vi "Base64 From Base64-URL.vi"(11 "Base64-URL String":string) -> (3 "Base64 String":string)   [LabVIEW 2018, in "Base64.lvlib"]
uses:
  Base64.lvlib
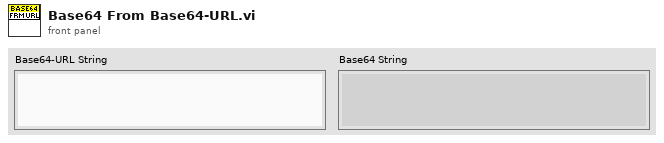
[diagram p1: front panel]
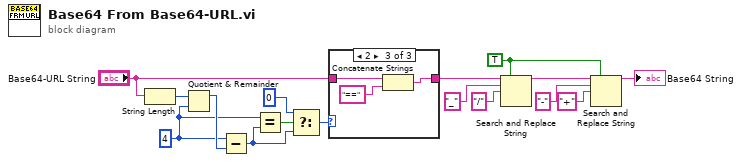
[diagram p0: block diagram]
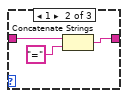
[diagram p3: hidden frame]
diagram:
  w3 = TRUE ("replace all? (F)")
  w14 = 4 ("y")
  n1 = String Length(string="Base64-URL String") -> (length=w16:i32)
  n2 = Quotient & Remainder(x=w16, y=w14) -> (x-y*floor(x/y)=w15:i32)  [unwired: 1 out]
  n3 = Subtract(x=w14, y=w15) -> (x-y=w12:i32)
  n4 = Equal?(x=w14, y=w12) -> (x = y?=w13:bool)
  n5 = Select(t=0, s=w13, f=w12) -> (s? t:f=w10:i32)
  n6 = case shown="2" w10 {
    tunnel: "Base64-URL String" -> [w17 w20 w23]
    tunnel: [w17 w18 w21] -> w2
    frame Default {
    }
    frame 1 {
      n7 = Concatenate Strings(w20, "=" ("string")) -> (w18:string)
    }
    frame 2 {
      n8 = Concatenate Strings(w23, "==" ("string")) -> (w21:string)
    }
  }
  n9 = Search and Replace String(replace all?=w3, input string=w2, search string="_", replace string="/" ("search string")) -> (result string=w4:string)  [unwired: 4 in, 3 out]
  n10 = Search and Replace String(replace all?=w3, input string=w4, search string="-", replace string="+" ("search string")) -> (result string=→"Base64 String":string)  [unwired: 4 in, 3 out]
